vi "Event from Ary I64.vi"(7 "Time Stamp":timestamp, 9 "Format":enum16{"Decimal", "Hexadecimal", "Binary"}(ring), 10 "Array":i64[](array[numeric]), 11 "VI Refnum":refnum<vi>) -> (2 "Event Data":T1)   [LabVIEW 2023, in "Instruments.lvlib" / "Instruments.lvclass"]
uses:
  Library/Instruments.lvclass
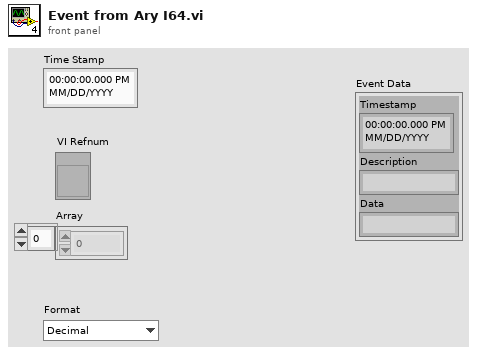
[diagram p1: front panel]
types:
  T1 = cluster{"Timestamp":timestamp, "Description":string, "Data":string}
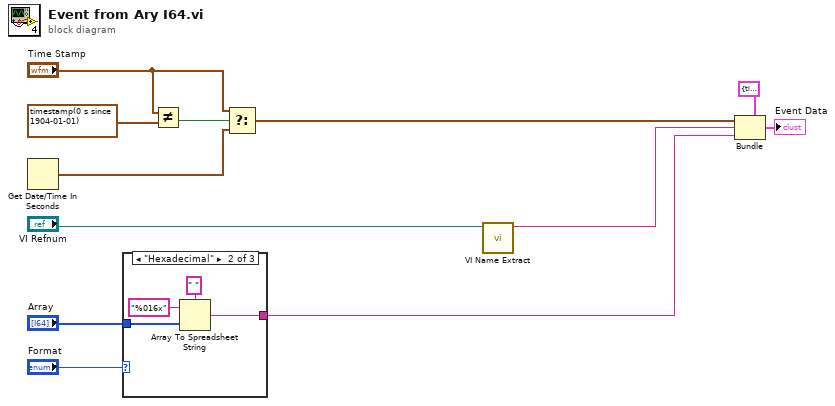
[diagram p0: block diagram]
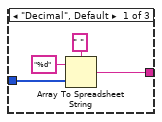
[diagram p2: hidden frame]
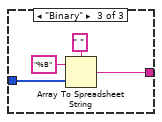
[diagram p3: hidden frame]
diagram:
  n1 = Get Date/Time In Seconds() -> (seconds since 1Jan1904=w5:timestamp)
  n2 = case shown="\"Hexadecimal\"" "Format" {
    tunnel: "Array" -> [w16 w20 w24]
    tunnel: [w15 w19 w23] -> w12
    frame "Decimal", Default {
      n3 = Array To Spreadsheet String(delimiter (Tab)=" ", array=w16, 3:"%d" ("format string")) -> (spreadsheet string=w15:string)
    }
    frame "Hexadecimal" {
      n4 = Array To Spreadsheet String(delimiter (Tab)=" ", array=w20, 3:"%016x" ("format string")) -> (spreadsheet string=w19:string)
    }
    frame "Binary" {
      n5 = Array To Spreadsheet String(delimiter (Tab)=" ", array=w24, 3:"%B" ("format string")) -> (spreadsheet string=w23:string)
    }
  }
  n6 = Not Equal?(x="Time Stamp", y=timestamp(0 s since 1904-01-01) ("Time Stamp")) -> (x != y?=w7:bool)
  n7 = Select(t="Time Stamp", s=w7, f=w5) -> (s? t:f=w4:timestamp)
  n8 = call "VI Name Extract.vi"("VI Refnum"="VI Refnum") -> ("Name"=w1:string)  [unwired: 10 in]
  n9 = Bundle(cluster=T1 {"Timestamp"=timestamp(0 s since 1904-01-01), "Description"="", "Data"=""}, "Timestamp"=w4, "Description"=w1, "Data"=w12) -> (→"Event Data":T1)
